vi "Jog Single Step.vi"(8 "error in (no error)":errorcluster, 10 "Jog Direction":T1, 11 "Thorlabs in":refnum<class "Thorlabs.lvclass">) -> (0 "error out":errorcluster, 3 "Thorlabs out":refnum<class "Thorlabs.lvclass">)   [LabVIEW 2018, in "Thorlabs.lvlib" / "Thorlabs.lvclass"]
doc: "Commands the Axis to jog the specified direction in a single step size."
uses:
  Thorlabs.lvclass
  PPLs/Axis/Parent/Axis.lvlibp/Custom Controls/Jog Direction.ctl
  PPLs/Axis/Parent/Axis.lvlibp
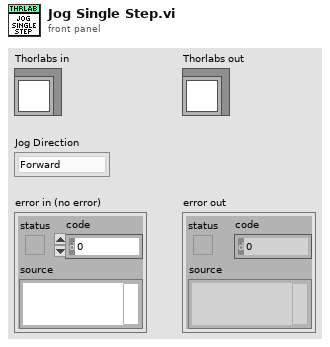
[diagram p1: front panel]
types:
  T1 = typedef "Axis.lvlibp/Jog Direction.ctl" = enum16{"Forward", "Backward"}
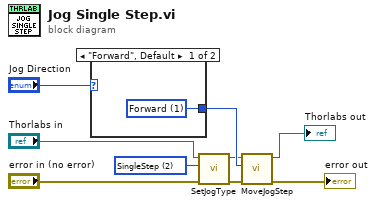
[diagram p0: block diagram]
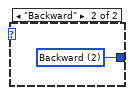
[diagram p2: hidden frame]
diagram:
  w1 = i16 2 items=["ContinuousHeld"=1, "SingleStep"=2, "ContinuousUnheld"=3] ("JogMode")
  n1 = case shown="\"Forward\", Default" "Jog Direction" {
    tunnel: [w10 w11] -> w7
    frame "Forward", Default {
      w10 = 1 items=["Forward"=1, "Backward"=2] ("direction")
    }
    frame "Backward" {
      w11 = 2 items=["Forward"=1, "Backward"=2] ("direction")
    }
  }
  n2 = call "SetJogType.vi"("Error In"="error in (no error)", "JogMode"=w1, "Thorlabs in"="Thorlabs in") -> ("Error Out"=w4:errorcluster, "Thorlabs out"=w2:refnum<class "Thorlabs.lvclass">)  [unwired: 7 in]
  n3 = call "MoveJogStep.vi"("Error In"=w4, "direction"=w7, "Thorlabs In"=w2) -> ("Error Out"=→"error out":errorcluster, "Thorlabs Out"=→"Thorlabs out":refnum<class "Thorlabs.lvclass">)  [unwired: 7 in]
